vi "List Available Captures for Timing Measurement.vi"(8 "error in (no error)":errorcluster, 10 "Timing measurement":string, 11 "Item Ref in":T1 format="%.0x") -> (0 "error out":errorcluster, 2 "captures available":string[](array[string]), 3 "Item Ref out":T1 format="%.0x")   [LabVIEW 2019, in "Engine Simulation Toolkit System Explorer.lvlib"]
uses:
  Engine Simulation Toolkit System Explorer.lvlib
  <vilib>/NI VeriStand/Custom Device API/Custom Device Item Ref.ctl
  Shared/Properties.vi
  Shared/Engine Simulation Toolkit Shared.lvlib
  <vilib>/NI VeriStand/Custom Device API/Custom Device API.lvlib
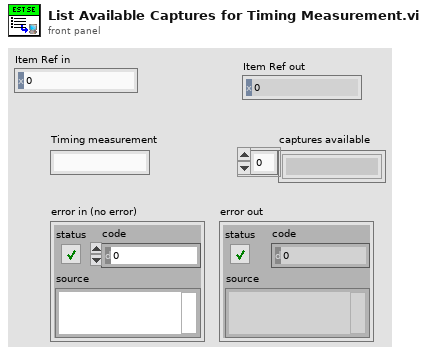
[diagram p1: front panel]
types:
  T1 = typedef "Custom Device API.lvlib/Custom Device Item Ref.ctl" = u64
  T2 = typedef "Custom Device API.lvlib/Custom Device Item Info.ctl" = cluster{"Name":string, "Is Channel":bool, "GUID":string, "Is Waveform":bool}
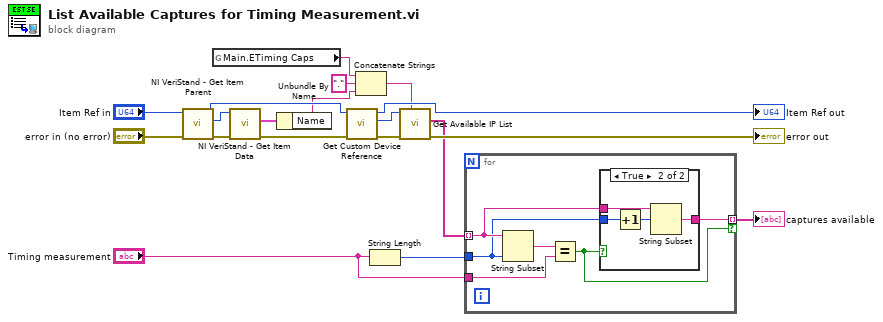
[diagram p0: block diagram]
diagram:
  n1 = call <vilib>:"NI VeriStand - Get Item Parent.vi"("error in (no error)"="error in (no error)", "Item Ref in"="Item Ref in") -> ("error out"=w9:errorcluster, "Parent Ref"=w8:T1, "Item Ref out"=w7:T1)  [unwired: 6 in, 1 out]
  n2 = global read "Properties.vi" "Main.ETiming Caps"() -> (w4:string)
  n3 = call <vilib>:"NI VeriStand - Get Item Data.vi"("error in (no error)"=w9, "Item Ref in"=w8) -> ("error out"=w6:errorcluster, "Item Info"=w3:T2)  [unwired: 6 in, 2 out]
  n4 = Unbundle By Name(w3) -> ("Name"=w2:string)
  n5 = call "Get Custom Device Reference.vi"("error in (no error)"=w6, "Item Ref in"=w7) -> ("error out"=w14:errorcluster, "Custom Device Ref"=w13:T1, "Item Ref out"=→"Item Ref out":T1)  [unwired: 7 in]
  n6 = Concatenate Strings(w4, "." ("string"), w2) -> (w1:string)
  n7 = String Length(string="Timing measurement") -> (length=w17:i32)
  n8 = call "Get Available IP List.vi"("ip list property name"=w1, "error in (no error)"=w14, "Item Ref in"=w13) -> ("error out"=→"error out":errorcluster, "ips available"=w18:string[])  [unwired: 6 in, 1 out]
  n9 = for {
    tunnel: w18 -> [w23] mode=indexing
    tunnel: w17 -> [w22]
    tunnel: "Timing measurement" -> [w24]
    tunnel: [w21] -> w15 mode=indexing if=w20
    n10 = String Subset(string=w23, length (rest)=w22) -> (substring=w25:string)  [unwired: 1 in]
    n11 = Equal?(x=w25, y=w24) -> (x = y?=w20:bool)
    n12 = case shown="True" w20 {
      tunnel: w23 -> [_ w29]
      tunnel: w22 -> [_ w27]
      tunnel: [_ w28] -> w21
      frame False {
      }
      frame True {
        n13 = Increment(x=w27) -> (x+1=w26:i32)
        n14 = String Subset(string=w29, offset (0)=w26) -> (substring=w28:string)  [unwired: 1 in]
      }
    }
  }
  "captures available" <- w15
